vi "Control_VI.vi"() -> ()   [LabVIEW 2026]
uses:
  <vilib>/Utility/miscctls.llb/LVPointTypeDef.ctl
  Control/Ctrl_GuiEvent.ctl
  Control/Ctrl_EscrituraComandos.ctl
panel:
  out "time string":string
  in  "Slid_muneca":i32(slide)=1 caption="SetPoint Muñeca (°)" scale=-45.0..45.0
  in  "PWM":dbl
  in  "Grabar":bool
  in  "Tabla":string[][](table)
  in  "Stop_moving":bool
  in  "Slid_hombro":i32(slide)=1 caption="Setpoint Hombro (°)" scale=-65.0..65.0
  in  "Play_button":bool
  in  "B_Home_Ind":bool
  in  "Ctrl_articulacion":T1(ring) caption="Control de la articulación"
  in  "Slid_gripper":i32(slide)=1 caption="Setpoint Gripper (Distancia)" scale=-90.0..90.0
  in  "Slid_antebrazo":i32(slide)=1 caption="SetPoint Antebrazo (°)" scale=-45.0..45.0
  in  "Slid_codo":i32(slide)=1 caption="Setpoint Codo (°)" scale=-55.0..55.0
  in  "Slid_cad":i32(slide)=1 caption="Setpoint Cadera (°)" scale=-150.0..150.0
  in  "B_abajo":bool
  in  "B_arriba":bool
  in  "B_der":bool
  in  "B_izq":bool
  # "Controles"
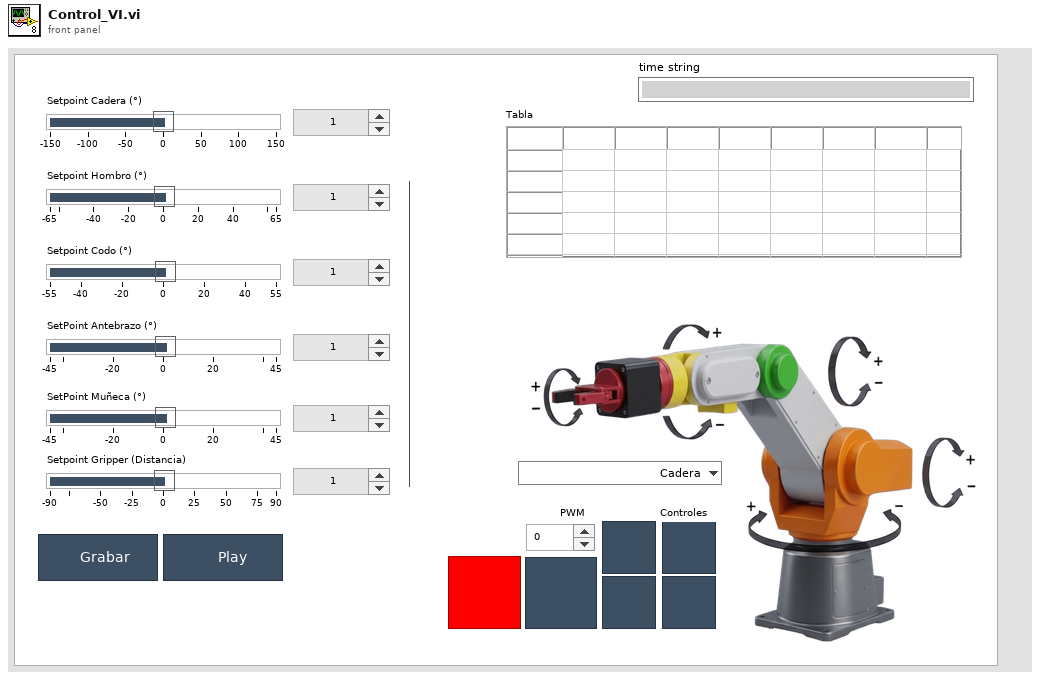
[diagram p1: front panel]
types:
  T1 = enum16{"Cadera", "Hombro", "Antebrazo", "Muñeca", "Gripper"}
  T2 = typedef "Ctrl_GuiEvent.ctl" = enum16{"Set Ref", "Update Enc", "Stop", "Get Ref"}
  T3 = typedef "LVPointTypeDef.ctl" = cluster{"Horizontal":i16, "Vertical":i16}
  T4 = cluster{"B_arriba":refnum<vi>, "B_izq":refnum<vi>, "B_der":refnum<vi>, "B_abajo":refnum<vi>, "Grabar":refnum<vi>, "Stop_moving":refnum<vi>, "Play_button":refnum<vi>, "B_Home_Ind":refnum<vi>, "Ctrl_articulacion":refnum<vi>, "Slid_cad":refnum<vi>, "Slid_hombro":refnum<vi>, "Slid_codo":refnum<vi>, "Slid_antebrazo":refnum<vi>, "Slid_gripper":refnum<vi>, "Tabla":refnum<vi>, "Slid_muneca":refnum<vi>}
  T5 = typedef "Ctrl_EscrituraComandos.ctl" = enum16{"GET REF", "SEND ESP32", "SET REF"}
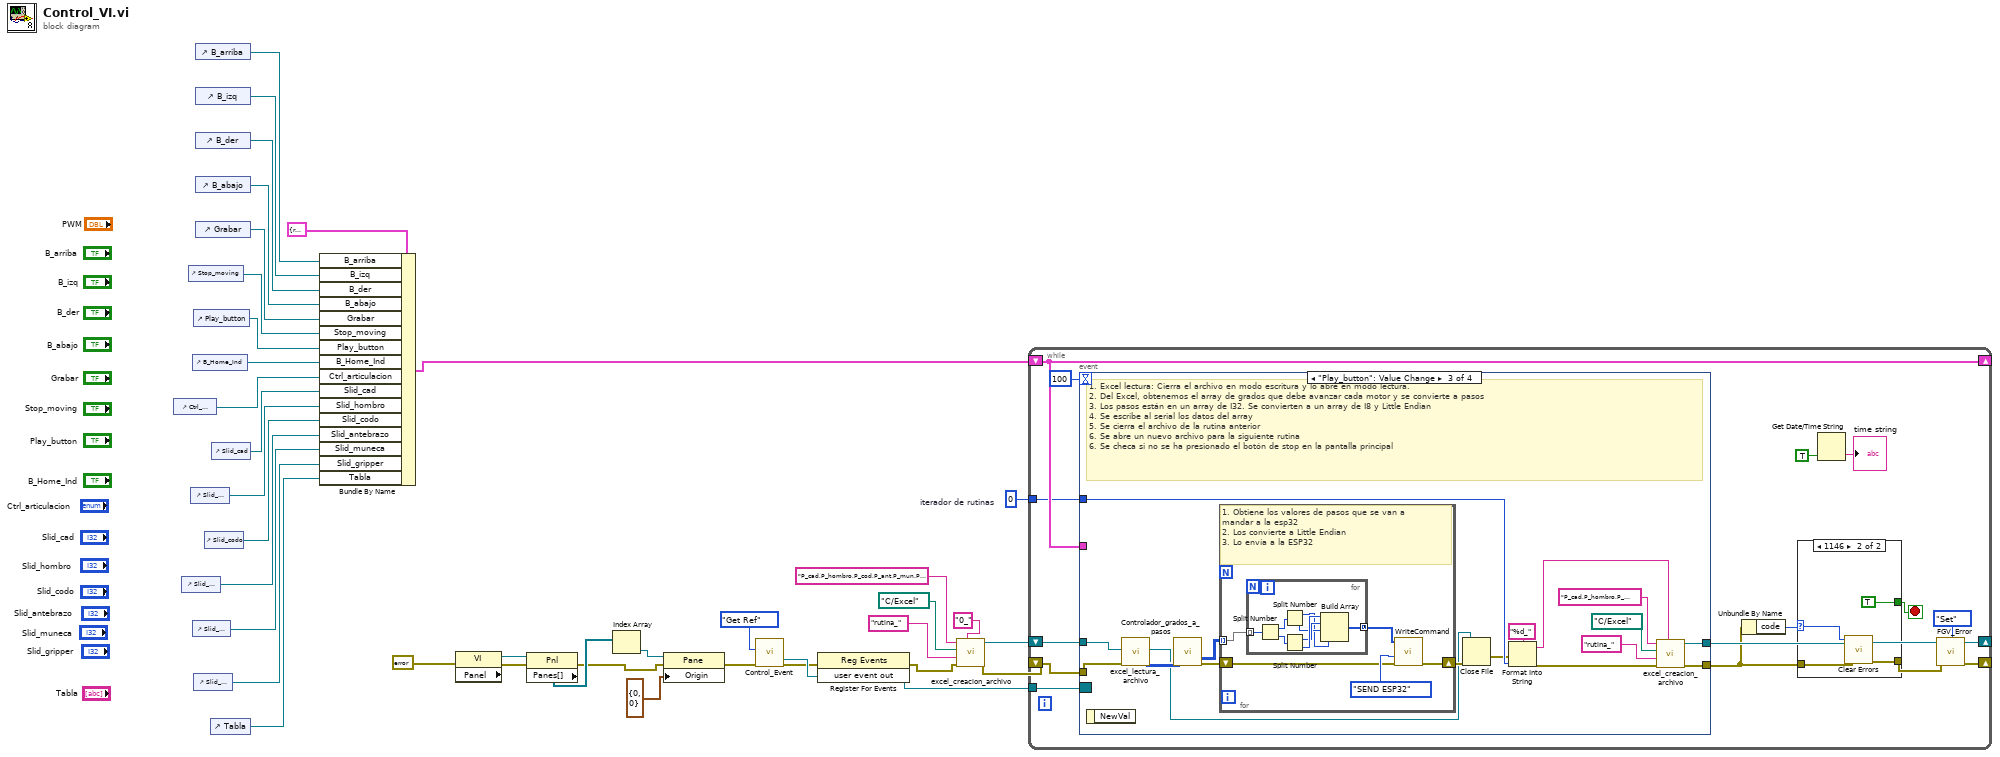
[diagram p0: block diagram]
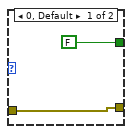
[diagram p2: hidden frame]
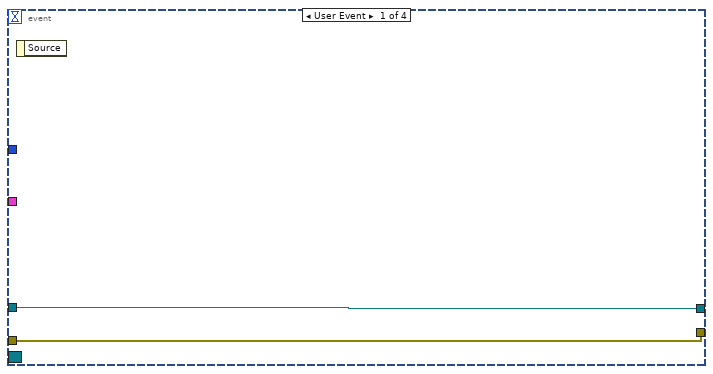
[diagram p3: hidden frame]
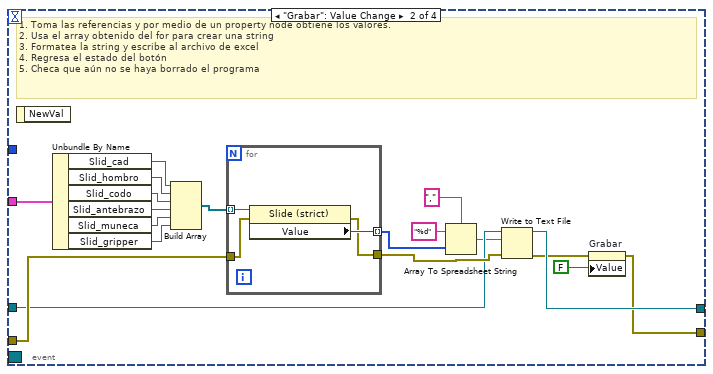
[diagram p4: hidden frame]
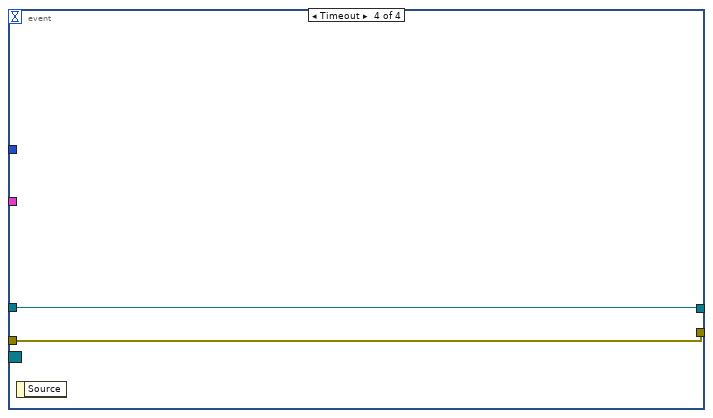
[diagram p5: hidden frame]
diagram:
  w1 = 0  # iterador de rutinas
  n1 = control-ref of="Ctrl_articulacion"() -> (w30:refnum<vi>)
  n2 = control-ref of="Slid_antebrazo"() -> (w26:refnum<vi>)
  n3 = control-ref of="Stop_moving"() -> (w33:refnum<vi>)
  n4 = control-ref of="Slid_hombro"() -> (w28:refnum<vi>)
  n5 = control-ref of="B_Home_Ind"() -> (w31:refnum<vi>)
  n6 = control-ref of="Slid_muneca"() -> (w2:refnum<vi>)
  n7 = control-ref of="Play_button"() -> (w32:refnum<vi>)
  n8 = control-ref of="Slid_gripper"() -> (w25:refnum<vi>)
  n9 = control-ref of="B_arriba"() -> (w38:refnum<vi>)
  n10 = control-ref of="B_izq"() -> (w37:refnum<vi>)
  n11 = control-ref of="B_der"() -> (w36:refnum<vi>)
  n12 = control-ref of="B_abajo"() -> (w35:refnum<vi>)
  n13 = control-ref of="Grabar"() -> (w34:refnum<vi>)
  n14 = control-ref of="Slid_codo"() -> (w27:refnum<vi>)
  n15 = control-ref of="Tabla"() -> (w24:refnum<vi>)
  n16 = control-ref of="Slid_cad"() -> (w29:refnum<vi>)
  n17 = Bundle By Name(cluster=T4 {"B_arriba"=refnum, "B_izq"=refnum, "B_der"=refnum, "B_abajo"=refnum, "Grabar"=refnum, "Stop_moving"=refnum, "Play_button"=refnum, "B_Home_Ind"=refnum, "Ctrl_articulacion"=refnum, "Slid_cad"=refnum, "Slid_hombro"=refnum, "Slid_codo"=refnum, "Slid_antebrazo"=refnum, "Slid_gripper"=refnum, "Tabla"=refnum, "Slid_muneca"=refnum}, "B_arriba"=w38, "B_izq"=w37, "B_der"=w36, "B_abajo"=w35, "Grabar"=w34, "Stop_moving"=w33, "Play_button"=w32, "B_Home_Ind"=w31, "Ctrl_articulacion"=w30, "Slid_cad"=w29, "Slid_hombro"=w28, "Slid_codo"=w27, "Slid_antebrazo"=w26, "Slid_muneca"=w2, "Slid_gripper"=w25, "Tabla"=w24) -> (w12:T4)
  n18 = property class="VI"(error in=errorcluster {"status"=FALSE, "code"=0, "source"=""} ("error out")) -> (error out=w21:errorcluster, "Panel"=w22:refnum<vi>)  [unwired: 1 in, 1 out]
  n19 = property class="Pnl"(reference=w22, error in=w21) -> (error out=w18:errorcluster, "Panes[]"=w20:refnum<vi>[])  [unwired: 1 out]
  n20 = Index Array(array=w20) -> (element=w19:refnum<vi>)  [unwired: 1 in]
  n21 = property class="Pane"(reference=w19, error in=w18, "Origin"=T3 {"Horizontal"=0, "Vertical"=0}) -> (error out=w6:errorcluster)  [unwired: 1 out]
  n22 = call "Control_Event.vi"("error in"=w6, "Estado"=Ctrl_GuiEvent."Get Ref") -> ("error out"=w5:errorcluster, "user event out"=w15:refnum<user-event>)  [unwired: 8 in]
  n23 = register-events(error in=w5, w15) -> (reference out=w13:refnum<event-registration>, error out=w11:errorcluster)  [unwired: 1 in]
  n24 = call "excel_creacion_archivo.vi"("número"="0_", "error in (no error)"=w11, "inicial archivo"="rutina_", "direccion carpeta"=path "C:/Excel" ("appended path"), "títulos columnas"="P_cad,P_hombro,P_cod,P_ant,P_mun,P_grip") -> ("error out"=w9:errorcluster, "Referencia Excel"=w8:refnum<file>)  [unwired: 5 in]
  n25 = while {
    tunnel: w13 -> [w53]
    shift-right: [w50] -> _
    shift-left: w9 -> [w51]
    shift-right: [w46] -> _
    shift-left: w12 -> [w46]
    shift-right: [w47] -> _
    shift-left: w8 -> [w48]
    tunnel: w1 -> [w42]
    stop <- w49 stop-if-true
    n26 = event shown="[2] \"Play_button\": Value Change" {
      selector: w53 -> [_ _ _ _]
      dyn-events: _ -> [_ _ _ _]
      timeout: 100 -> [_ _ _ _]
      tunnel: w51 -> [w60 w72 w102 w117]
      tunnel: [w60 w62 w96 w117] -> w45
      tunnel: w46 -> [_ w79 _ _]
      tunnel: w48 -> [w61 w67 w101 w116]
      tunnel: [w61 w66 w88 w116] -> w47
      tunnel: w42 -> [_ _ w91 _]
      event User Event {
        n27 = event-data() -> ()  [unwired: 1 in, 1 out]
      }
      event "Grabar": Value Change {
        # "1. Toma las referencias y por medio de un property node obtiene los valores.\n2. Usa el array obtenido del for para crear una string\n3. Formatea la string y escribe al archivo de excel\n4. Regresa el estado del botón\n5. Checa que aún no se haya borrado el programa"
        n28 = event-data() -> ()  [unwired: 1 in, 1 out]
        n29 = Unbundle By Name(w79) -> ("Slid_cad"=w64:refnum<vi>, "Slid_hombro"=w78:refnum<vi>, "Slid_codo"=w77:refnum<vi>, "Slid_antebrazo"=w76:refnum<vi>, "Slid_muneca"=w75:refnum<vi>, "Slid_gripper"=w74:refnum<vi>)
        n30 = Build Array(w64, w78, w77, w76, w75, w74) -> (w73:refnum<vi>[])
        n31 = for {
          tunnel: w73 -> [w84] mode=indexing
          tunnel: w72 -> [w83]
          tunnel: [w82] -> w71 mode=indexing
          tunnel: [w81] -> w68
          n32 = property class="Slide (strict)"(reference=w84, error in=w83) -> (error out=w81:errorcluster, "Value"=w82:i32)  [unwired: 1 out]
        }
        n33 = Array To Spreadsheet String(delimiter (Tab)=",", array=w71, 3:"%d" ("format string")) -> (spreadsheet string=w63:string)
        n34 = Write to Text File(file (use dialog)=w67, text=w63, error in=w68) -> (refnum out=w66:refnum<file>, error out=w65:errorcluster)  [unwired: 1 in, 1 out]
        n35 = property on="Grabar" class="Bool (strict)"(error in=w65, "Value"=FALSE) -> (error out=w62:errorcluster)  [unwired: 1 in, 1 out]
      }
      event "Play_button": Value Change {
        # "1. Excel lectura: Cierra el archivo en modo escritura y lo abre en modo lectura.\n2. Del Excel, obtenemos el array de grados que debe avanzar cada motor y se convierte a pasos\n3. Los pasos están en un array de I32. Se convierten a un array de I8 y Little Endian\n4. Se escribe al serial los datos del array\n5. Se cierra el archivo de la rutina anterior\n6. Se abre un nuevo archivo para la siguiente rutina\n6. Se checa si no se ha presionado el botón de stop en la pantalla principal"
        n36 = event-data() -> ()  [unwired: 1 in, 1 out]
        n37 = call "excel_lectura_archivo.vi"("error in (no error)"=w102, "referencia excel in"=w101) -> ("error out"=w99:errorcluster, "array_grados"=w100:i64[][], "referencia excel out"=w85:refnum<file>)  [unwired: 6 in, 1 out]
        n38 = call "Controlador_grados_a_pasos.vi"("error in (no error)"=w99, "array_grados"=w100) -> ("error in (no error) 2"=w97:errorcluster, "array_pasos"=w98:i32[][])  [unwired: 8 in]
        n39 = for {
          tunnel: w98 -> [w104] mode=indexing
          shift-right: [w105] -> w87
          shift-left: w97 -> [w106]
          # "1. Obtiene los valores de pasos que se van a mandar a la esp32\n2. Los convierte a Little Endian\n3. Lo envía a la ESP32"
          n40 = for {
            tunnel: w104 -> [w115] mode=indexing
            tunnel: [w108] -> w103 mode=concatenating
            n41 = Split Number(x=w115) -> (hi(x)=w113:u16, lo(x)=w114:u16)
            n42 = Split Number(x=w113) -> (hi(x)=w109:u8, lo(x)=w110:u8)
            n43 = Split Number(x=w114) -> (hi(x)=w111:u8, lo(x)=w112:u8)
            n44 = Build Array(w112, w111, w110, w109) -> (w108:u8[])
          }
          n45 = call "WriteCommand.vi"("error in"=w106, "Com_Escribir"=Ctrl_EscrituraComandos."SEND ESP32", "Array_u8"=w103) -> ("error out"=w105:errorcluster)  [unwired: 7 in, 1 out]
        }
        n46 = Close File(refnum=w85, error in=w87) -> (error out=w86:errorcluster)  [unwired: 1 out]
        n47 = Format Into String(format string="%d_", error in=w86, w91) -> (resulting string=w92:string, error out=w89:errorcluster)  [unwired: 1 in]
        n48 = call "excel_creacion_archivo.vi"("número"=w92, "error in (no error)"=w89, "inicial archivo"="rutina_", "direccion carpeta"=path "C:/Excel" ("appended path"), "títulos columnas"="P_cad,P_hombro,P_cod,P_ant,P_mun,P_grip") -> ("error out"=w96:errorcluster, "Referencia Excel"=w88:refnum<file>)  [unwired: 5 in]
      }
      event Timeout {
        n49 = event-data() -> ()  [unwired: 1 in, 1 out]
      }
    }
    n50 = Unbundle By Name(w45) -> ("code"=w44:i32)
    n51 = case shown="1146" w44 {
      selector: w44 -> [_ w59]
      tunnel: [FALSE TRUE] -> w49
      tunnel: w45 -> [w54 w57]
      tunnel: [w54 w56] -> w43
      frame 0, Default {
      }
      frame 1146 {
        n52 = call <vilib>:"Clear Errors.vi"("error in (no error)"=w57, "specific error code to clear (0: all)"=w59) -> ("error out"=w56:errorcluster)  [unwired: 4 in, 1 out]
      }
    }
    n53 = Get Date/Time String(want seconds? (F)=TRUE) -> (time string=→"time string":string)  [unwired: 2 in, 1 out]
    n54 = call "FGV_Error.vi"("error_in_loop"=w43, "Estado"=enum16{"Set", "Get"}."Set") -> ("error out"=w50:errorcluster)  [unwired: 9 in]
  }
